vi "MTec_Init.vi"(0 "object in":refnum<class "MTec.lvclass">, 5 "error in (no error)":errorcluster) -> (14 "object out":refnum<class "MTec.lvclass">, 19 "error out":errorcluster)   [LabVIEW 2019, in "MTec.lvclass"]
uses:
  MTec.lvclass
  TEC LabVIEW Control Software v0.14/Source/LV Source/Variables/FGVs/Type Defs/FGV_Operations.ctl
  TEC LabVIEW Control Software v0.14/Source/LV Source/[meerstetter engineering TE Cooling]/TypeDefs/meTEC_Configuration.ctl
  MTec.lvclass/MTec.ctl
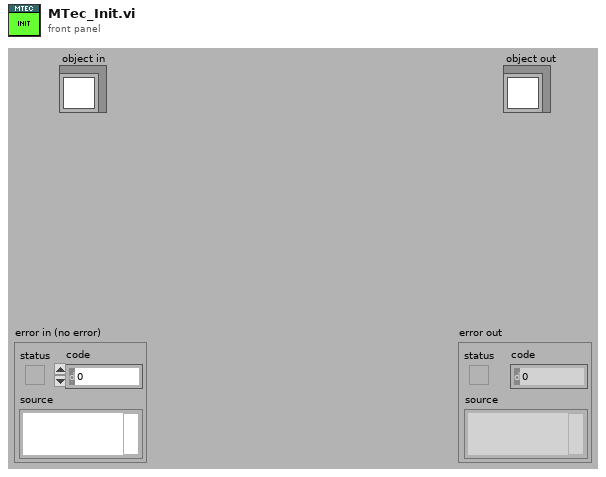
[diagram p1: front panel]
types:
  T1 = typedef "FGV_Operations.ctl" = enum16{"Read", "Write"}
  T2 = typedef "meTEC_Configuration.ctl" = cluster{"VISA resource name":refnum<visa-resource-name>, "Device Address":u16}
  T3 = typedef "FGV_TE Controller.ctl" = cluster{"SVs":cluster{"Unused":dbl}, "PVs":cluster{"FW & HW Versions":cluster{"Device Type [I32]":i32, "Device Type [String]":string, "Firmware Version [I32]":i32, "Firmware Version [String]":string, "Hardware Version [I32]":i32, "Hardware Version [String]":string, "Serial No.":i32}, "TEC Configuration":T2, "Object Target Temperature Source_CH1":u8, "Object Target Temperature Source_CH2":u8}, "Front Panel References":T4}
  T4 = typedef "FGV_Front Panel References.ctl" = cluster{"Main Loop Queue":refnum<queue>, "meTEC_Device Type":refnum<vi>, "meTEC_Serial No.":refnum<vi>, "meTEC_Hardware Version":refnum<vi>, "meTEC_Firmware Version":refnum<vi>, "meTEC_CH1_Object Target Temperature (ID 3000 / 50012) [°C]":refnum<vi>, "meTEC_CH1_Live Set Current (ID 50001) [A]":refnum<vi>, "meTEC_CH1_Live Set Voltage (ID 50002) [V]":refnum<vi>, "meTEC_CH1_Live Enable (ID 50000)":refnum<vi>, "meTEC_CH1_Input Selection (ID 2000)":refnum<vi>, "meTEC_CH1_Object Target Temp. Source Sel. (ID 50011)":refnum<vi>, "meTEC_CH2_Object Target Temperature (ID 3000 / 50012) [°C]":refnum<vi>, "meTEC_CH2_Live Set Current (ID 50001) [A]":refnum<vi>, "meTEC_CH2_Live Set Voltage (ID 50002) [V]":refnum<vi>, "meTEC_CH2_Live Enable (ID 50000)":refnum<vi>, "meTEC_CH2_Input Selection (ID 2000)":refnum<vi>, "meTEC_CH2_Object Target Temp. Source Sel. (ID 50011)":refnum<vi>, "meTEC_CH2_Object Temperature [°C]":refnum<vi>, "meTEC_CH2_Sink Temperature [°C]":refnum<vi>, "meTEC_CH2_Act. Output Current [A]":refnum<vi>, "meTEC_CH2_Act. Output Voltage [V]":refnum<vi>, "meTEC_CH2_Temperature Stability":refnum<vi>, "Monitor Chart_CH2":refnum<vi>, "meTEC_Initialize Device":refnum<vi>}
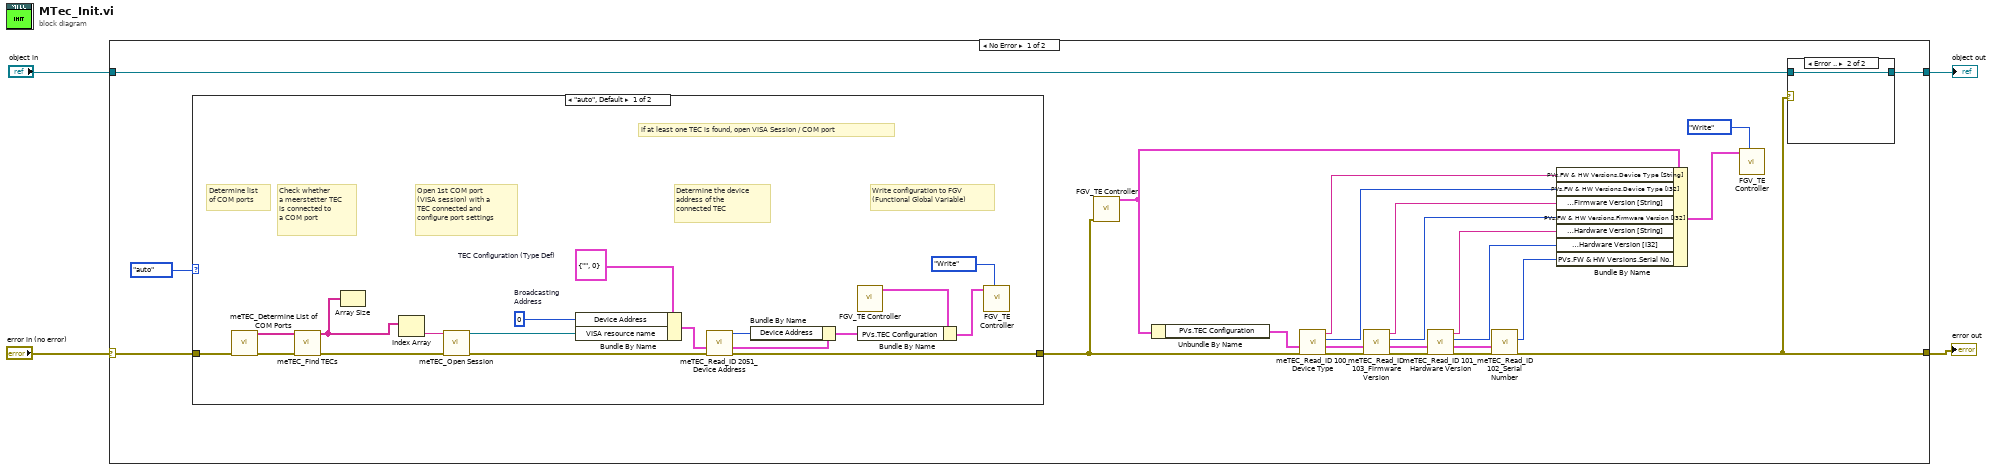
[diagram p0: block diagram]
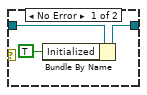
[diagram p2: hidden frame]
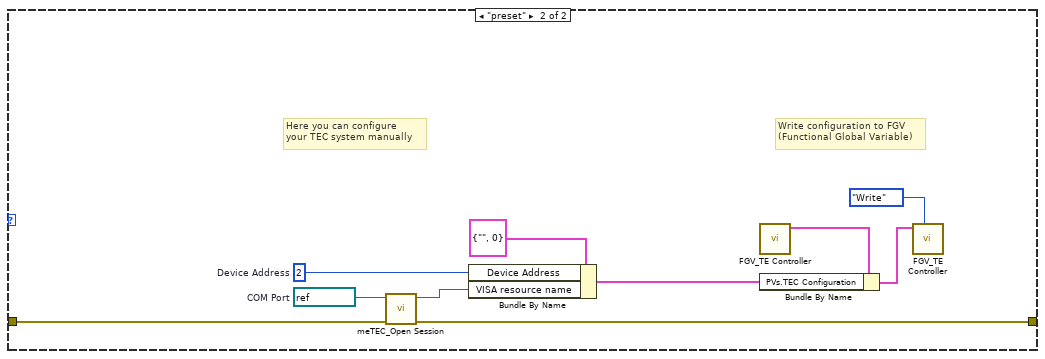
[diagram p3: hidden frame]
diagram:
  n1 = case shown="No Error" "error in (no error)" {
    selector: "error in (no error)" -> [w9 w60]
    tunnel: "object in" -> [w8 w61]
    tunnel: [w6 w61] -> w3
    tunnel: [w5 w60] -> w1
    frame No Error {
      n2 = case shown="\"auto\", Default" enum16{"auto", "preset"}."auto" {
        tunnel: w9 -> [w46 w55]
        tunnel: [w32 w50] -> w7
        frame "auto", Default {
          w44 = T2 {"VISA resource name"="", "Device Address"=0}  # TEC Configuration (Type Def)
          w43 = u16 0  # Broadcasting  Address
          # "Write configuration to FGV\n(Functional Global Variable)"
          # "Determine the device\naddress of the \nconnected TEC"
          # "Open 1st COM port\n(VISA session) with a\nTEC connected and\nconfigure port settings"
          # "if at least one TEC is found, open VISA Session / COM port"
          # "Check whether\na meerstetter TEC\nis connected to\na COM port"
          # "Determine list\nof COM ports"
          n3 = call "meTEC_Determine List of COM Ports.vi"("error in (no error)"=w46) -> ("error out"=w49:errorcluster, "VISA Resources List (COM Ports)"=w48:string[])  [unwired: 9 in]
          n4 = call "meTEC_Find TECs.vi"("error in (no error)"=w49, "VISA Resources List (COM Ports)"=w48) -> ("error out"=w47:errorcluster, "VISA Resources List (meTEC(s))"=w45:string[])  [unwired: 8 in]
          n5 = Array Size(array=w45) -> ()  [unwired: 1 out]
          n6 = Index Array(array=w45) -> (element=w33:string)  [unwired: 1 in]
          n7 = call "meTEC_Open Session.vi"("error in (no error)"=w47, "COM Port"=w33) -> ("error out"=w42:errorcluster, "VISA resource name_OUT"=w41:refnum<visa-resource-name>)  [unwired: 8 in]
          n8 = Bundle By Name(cluster=w44, "Device Address"=w43, "VISA resource name"=w41) -> (w40:T2)
          n9 = call "meTEC_Read_ID 2051_Device Address.vi"("error in (no error)"=w42, "TEC Configuration_IN"=w40) -> ("error out"=w32:errorcluster, "TEC Configuration_OUT"=w38:T2, "Device Address (ID 2051) [I32]"=w39:i32)  [unwired: 7 in]
          n10 = Bundle By Name(cluster=w38, "Device Address"=w39) -> (w34:T2)
          n11 = call "FGV_TE Controller.vi"() -> ("FGV_TEC_OUT"=w37:T3)  [unwired: 10 in, 1 out]
          n12 = Bundle By Name(cluster=w37, "PVs.TEC Configuration"=w34) -> (w36:T3)
          n13 = call "FGV_TE Controller.vi"("Operation (Read)"=FGV_Operations."Write", "FGV_TEC_IN"=w36) -> ()  [unwired: 8 in, 2 out]
        }
        frame "preset" {
          w57 = u16 2  # Device Address
          w59 = refnum<visa-resource-name> "COM4"  # COM Port
          # "Here you can configure\nyour TEC system manually"
          # "Write configuration to FGV\n(Functional Global Variable)"
          n14 = call "meTEC_Open Session.vi"("error in (no error)"=w55, "COM Port"=w59) -> ("error out"=w50:errorcluster, "VISA resource name_OUT"=w56:refnum<visa-resource-name>)  [unwired: 8 in]
          n15 = Bundle By Name(cluster=T2 {"VISA resource name"="", "Device Address"=0} ("TEC Configuration"), "Device Address"=w57, "VISA resource name"=w56) -> (w51:T2)
          n16 = call "FGV_TE Controller.vi"() -> ("FGV_TEC_OUT"=w54:T3)  [unwired: 10 in, 1 out]
          n17 = Bundle By Name(cluster=w54, "PVs.TEC Configuration"=w51) -> (w53:T3)
          n18 = call "FGV_TE Controller.vi"("Operation (Read)"=FGV_Operations."Write", "FGV_TEC_IN"=w53) -> ()  [unwired: 8 in, 2 out]
        }
      }
      n19 = call "FGV_TE Controller.vi"("error in (no error)"=w7) -> ("FGV_TEC_OUT"=w22:T3)  [unwired: 9 in, 1 out]
      n20 = Unbundle By Name(w22) -> ("PVs.TEC Configuration"=w21:T2)
      n21 = call "meTEC_Read_ID 100_Device Type.vi"("error in (no error)"=w7, "TEC Configuration_IN"=w21) -> ("error out"=w25:errorcluster, "TEC Configuration_OUT"=w20:T2, "Device Type (ID 100) [I32]"=w11:i32, "Device Type (ID 100) [String]"=w12:string)  [unwired: 6 in]
      n22 = call "meTEC_Read_ID 103_Firmware Version.vi"("error in (no error)"=w25, "TEC Configuration_IN"=w20) -> ("error out"=w24:errorcluster, "TEC Configuration_OUT"=w19:T2, "Firmware Version (ID 103) [I32]"=w13:i32, "Firmware Version (ID 103) [String]"=w14:string)  [unwired: 6 in]
      n23 = call "meTEC_Read_ID 101_Hardware Version.vi"("error in (no error)"=w24, "TEC Configuration_IN"=w19) -> ("error out"=w23:errorcluster, "TEC Configuration_OUT"=w18:T2, "Hardware Version (ID 101) [I32]"=w15:i32, "Hardware Version (ID 101) [String]"=w16:string)  [unwired: 6 in]
      n24 = call "meTEC_Read_ID 102_Serial Number.vi"("error in (no error)"=w23, "TEC Configuration_IN"=w18) -> ("error out"=w5:errorcluster, "Serial No. (ID 102) [I32]"=w17:i32)  [unwired: 6 in, 2 out]
      n25 = Bundle By Name(cluster=w22, "PVs.FW & HW Versions.Device Type [String]"=w12, "PVs.FW & HW Versions.Device Type [I32]"=w11, "PVs.FW & HW Versions.Firmware Version [String]"=w14, "PVs.FW & HW Versions.Firmware Version [I32]"=w13, "PVs.FW & HW Versions.Hardware Version [String]"=w16, "PVs.FW & HW Versions.Hardware Version [I32]"=w15, "PVs.FW & HW Versions.Serial No."=w17) -> (w27:T3)
      n26 = call "FGV_TE Controller.vi"("Operation (Read)"=FGV_Operations."Write", "FGV_TEC_IN"=w27) -> ()  [unwired: 8 in, 2 out]
      n27 = case shown="Error .." w5 {
        tunnel: w8 -> [w30 w31]
        tunnel: [w29 w31] -> w6
        frame No Error {
          n28 = Bundle By Name(cluster=w30, "Initialized"=TRUE) -> (w29:refnum<class "MTec.lvclass">)
        }
        frame Error {
        }
      }
    }
    frame Error {
    }
  }
  "object out" <- w3
  "error out" <- w1
